vi "SecondsToTimeStamp.vi"(1 "Time [s]":dbl format="%#_13g") -> (0 "TimeStamp":string)   [LabVIEW 2015]
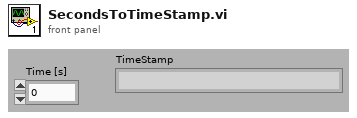
[diagram p1: front panel]
types:
  T1 = typedef "LVDateTimeRec.ctl" = cluster{"fractional second":dbl, "second":i32, "minute":i32, "hour":i32, "day of month":i32, "month":i32, "year":i32, "day of week":i32, "day of year":i32, "DST":i32}
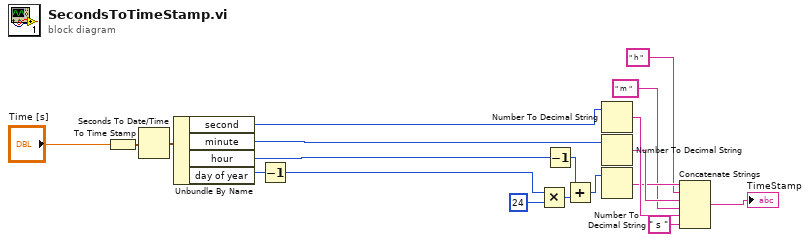
[diagram p0: block diagram]
diagram:
  n1 = To Time Stamp(1:"Time [s]") -> (0:w15:timestamp)
  n2 = Seconds To Date/Time(time stamp (now)=w15) -> (date time rec=w16:T1)  [unwired: 1 in]
  n3 = Unbundle By Name(w16) -> ("second"=w10:i32, "minute"=w9:i32, "hour"=w8:i32, "day of year"=w6:i32)
  n4 = Decrement(x=w6) -> (x-1=w5:i32)
  n5 = Multiply(x=w5, y=24) -> (x*y=w11:i32)
  n6 = Decrement(x=w8) -> (x-1=w13:i32)
  n7 = Add(x=w13, y=w11) -> (x+y=w12:i32)
  n8 = Number To Decimal String(number=w10) -> (decimal integer string=w19:string)  [unwired: 1 in]
  n9 = Number To Decimal String(number=w9) -> (decimal integer string=w18:string)  [unwired: 1 in]
  n10 = Number To Decimal String(number=w12) -> (decimal integer string=w17:string)  [unwired: 1 in]
  n11 = Concatenate Strings(w17, " h " ("string"), w18, " m " ("string"), w19, " s " ("string")) -> (→"TimeStamp":string)
